vi "Polling.vi"(8 "error in (no error)":errorcluster, 11 "Node Ptr":T1 format="%.0x") -> (0 "error out":errorcluster)   [LabVIEW 2019, in "Diagnostics Addon System Explorer.lvlib"]
uses:
  Diagnostics Addon System Explorer.lvlib
  <vilib>/NI VeriStand/Custom Device API/Custom Device Item Ref.ctl
  Types/FG.Action.ctl
  Addon Shared/SubVIs/Constants.vi
  <vilib>/NI VeriStand/Custom Device API/Custom Device API.lvlib
panel:
  in  "SHDocVw.IWebBrowser":refnum<k7>(container)
  in  "Collection":i32(listbox) caption="Items"
  in  "Description":string
  out "Name":string
  in  "Header":cluster{"Section Name":string}={"Section Name"="Custom Device Item Settings"}
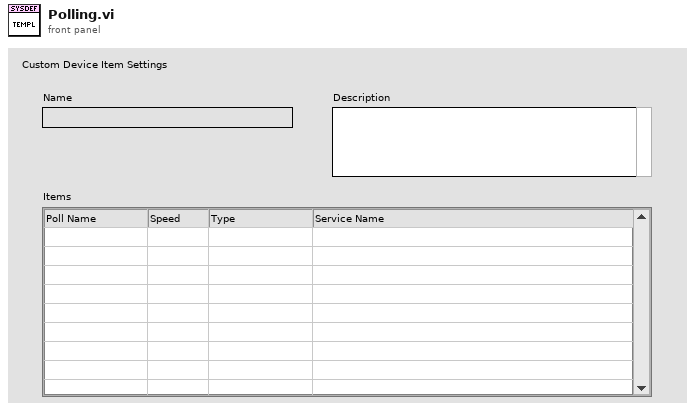
[diagram p1: front panel]
types:
  T1 = typedef "Custom Device API.lvlib/Custom Device Item Ref.ctl" = u64
  T2 = typedef "Diagnostics Addon System Explorer.lvlib/FG.Action.ctl" = enum16{"Get", "Set"}
  T3 = typedef "Custom Device API.lvlib/Custom Device Item Info.ctl" = cluster{"Name":string, "Is Channel":bool, "GUID":string, "Is Waveform":bool}
  T4 = typedef "Diagnostics Addon System Explorer.lvlib/Poll.Settings.ctl" = cluster{"Input Channels":T5[], "Speed":T6}
  T5 = typedef "Diagnostics Addon System Explorer.lvlib/Poll.LinkedNode.ctl" = cluster{"Node ID":u64}
  T6 = typedef "Diagnostics Addon Shared.lvlib/DPID.Rate.ctl" = enum16{"Slow", "Medium", "Fast"}
  T7 = typedef "Custom Device API.lvlib/Custom Device Commands.ctl" = enum16{"Default", "Item renamed", "Shutdown", "Dynamic button pressed"}
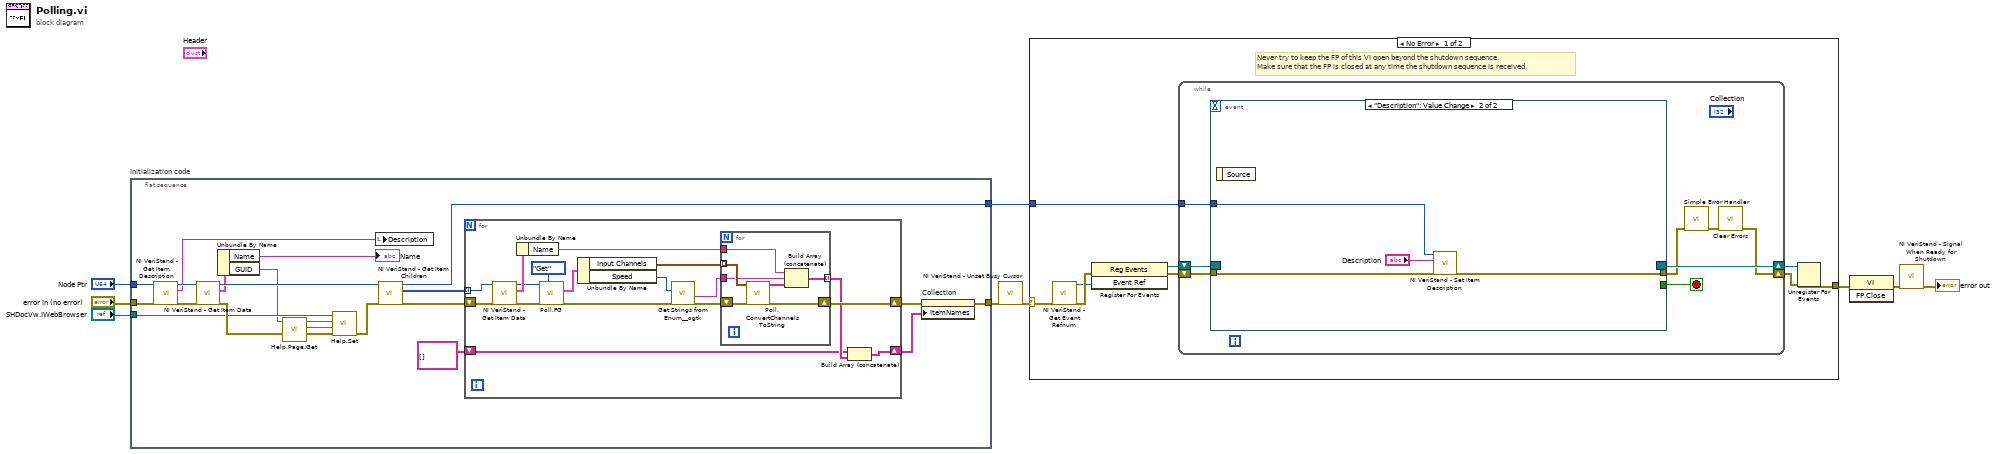
[diagram p0: block diagram]
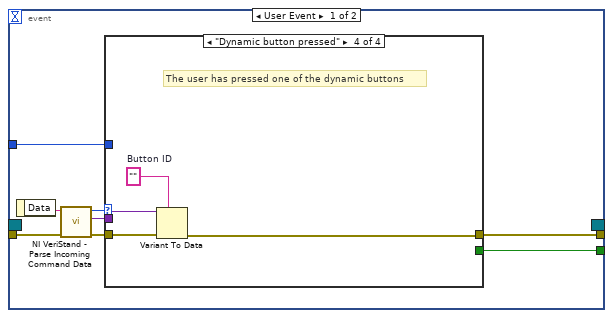
[diagram p2: hidden frame]
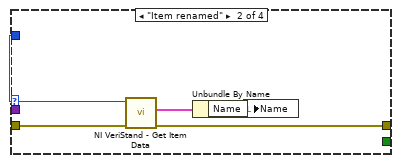
[diagram p4: hidden frame]
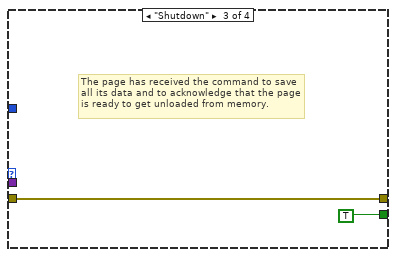
[diagram p5: hidden frame]
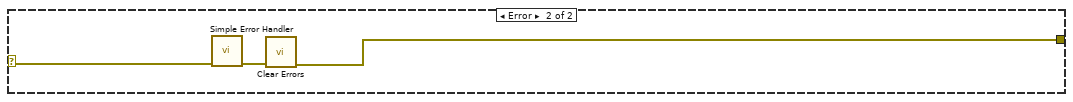
[diagram p6: hidden frame]
diagram:
  n1 = flat-sequence "Initialization code" {
    tunnel: "error in (no error)" -> [w15]
    tunnel: [w20] -> w6
    tunnel: [w22] -> w3
    tunnel: "Node Ptr" -> [w25]
    tunnel: "SHDocVw.IWebBrowser" -> [w16]
    frame #0 {
      n2 = call <vilib>:"NI VeriStand - Get Item Description.vi"("error in (no error)"=w15, "Item Ref in"=w25) -> ("error out"=w27:errorcluster, "Description"=w28:string, "Item Ref out"=w29:T1)  [unwired: 7 out]
      n3 = call <vilib>:"NI VeriStand - Get Item Data.vi"("error in (no error)"=w27, "Item Ref in"=w29) -> ("error out"=w18:errorcluster, "Item Info"=w26:T3, "Item Ref out"=w30:T1)  [unwired: 7 out]
      n4 = Unbundle By Name(w26) -> ("Name"=→"Name":string, "GUID"=w12:string)
      n5 = call "Help.Page.Get.vi"("GUID"=w12) -> ("HTML File"=w11:string, "Main CHM File"=w10:string)  [unwired: 9 in]
      n6 = call "Help.Set.vi"("error in (no error)"=w18, "HTML File"=w11, "Main CHM File"=w10, "SHDocVw.IWebBrowser2"=w16) -> ("error out"=w17:errorcluster)  [unwired: 7 in]
      n7 = local write "Description"(w28) -> ()
      n8 = call <vilib>:"NI VeriStand - Get Item Children.vi"("error in (no error)"=w17, "Item Ref in"=w30) -> ("error out"=w24:errorcluster, "Child Refs"=w23:T1[], "Item Ref out"=w22:T1)  [unwired: 6 in, 1 out]
      n9 = for {
        shift-right: [w40] -> w21
        shift-left: w24 -> [w46]
        tunnel: w23 -> [w45] mode=indexing
        shift-right: [w37] -> w14
        shift-left: string[][] [] -> [w36]
        n10 = call <vilib>:"NI VeriStand - Get Item Data.vi"("error in (no error)"=w46, "Item Ref in"=w45) -> ("error out"=w42:errorcluster, "Item Info"=w47:T3, "Item Ref out"=w41:T1)  [unwired: 7 out]
        n11 = Unbundle By Name(w47) -> ("Name"=w39:string)
        n12 = call "Poll.FG.vi"("Action"=FG.Action."Get", "error in"=w42, "Parent Ref"=w41) -> ("error out"=w35:errorcluster, "Selected Channels out"=w43:T4)  [unwired: 6 in, 1 out]
        n13 = Unbundle By Name(w43) -> ("Input Channels"=w31:T5[], "Speed"=w33:T6)
        n14 = call <userlib>:"Get Strings from Enum__ogtk.vi"("error in (no error)"=w35, "Enum"=w33) -> ("error out"=w34:errorcluster, "String Value"=w32:string)  [unwired: 6 in, 2 out]
        n15 = for {
          shift-right: [w52] -> w40
          shift-left: w34 -> [w54]
          tunnel: w31 -> [w53] mode=indexing
          tunnel: [w49] -> w38 mode=indexing
          tunnel: w39 -> [w51]
          tunnel: w32 -> [w48]
          n16 = call "Poll.ConvertChannelsToString.vi"("error in (no error)"=w54, "MonitoredChannelSettings"=w53) -> ("error out"=w52:errorcluster, "Array"=w50:string[])  [unwired: 8 in]
          n17 = Build Array (concatenate)(w51, w48, w50) -> (w49:string[])
        }
        n18 = Build Array (concatenate)(w36, w38) -> (w37:string[][])
      }
      n19 = property on="Collection" class="MCListbox (strict)"(error in=w21, "ItemNames"=w14) -> (error out=w20:errorcluster)  [unwired: 1 in, 1 out]
    }
  }
  n20 = call <vilib>:"NI VeriStand - Unset Busy Cursor.vi"("error in (no error)"=w6) -> ("error out"=w5:errorcluster)  [unwired: 10 out]
  n21 = case shown="No Error" w5 {
    selector: w5 -> [w55 w98]
    tunnel: [w60 w96] -> w9
    tunnel: w3 -> [w56 _]
    frame No Error {
      # "Never try to keep the FP of this VI open beyond the shutdown sequence.\nMake sure that the FP is closed at any time the shutdown sequence is received."
      n22 = call <vilib>:"NI VeriStand - Get Event Refnum.vi"("error in (no error)"=w55) -> ("error out"=w63:errorcluster, "Event Ref"=w59:refnum<user-event>)  [unwired: 9 out]
      n23 = register-events(error in=w63, w59) -> (reference out=w57:refnum<event-registration>, error out=w58:errorcluster)  [unwired: 1 in]
      n24 = while {
        tunnel: w56 -> [w67]
        shift-right: [w64] -> w61
        shift-left: w58 -> [w70]
        shift-right: [w71] -> w62
        shift-left: w57 -> [w69]
        stop <- w68 stop-if-true
        n25 = event shown="[1] \"Description\": Value Change" {
          selector: w69 -> [_ _]
          dyn-events: [_ _] -> w71
          timeout: _ -> [_ _]
          tunnel: w70 -> [w79 w94]
          tunnel: [w75 _] -> w68
          tunnel: [w74 w93] -> w66
          tunnel: w67 -> [w73 w95]
          event User Event {
            n26 = event-data() -> ("Data"=w78:string)  [unwired: 1 out]
            n27 = call <vilib>:"NI VeriStand - Parse Incoming Command Data.vi"("error in (no error)"=w79, "Incoming data"=w78) -> ("error out"=w77:errorcluster, "Outgoing data"=w72:variant, "Action"=w76:T7)  [unwired: 7 out]
            n28 = case shown="\"Dynamic button pressed\"" w76 {
              tunnel: w77 -> [w80 w85 w86 w91]
              tunnel: [_ _ TRUE _] -> w75
              tunnel: [w80 w82 w86 w88] -> w74
              tunnel: w73 -> [_ w84 _ _]
              tunnel: w72 -> [_ _ _ w90]
              frame "Default", Default {
              }
              frame "Item renamed" {
                n29 = call <vilib>:"NI VeriStand - Get Item Data.vi"("error in (no error)"=w85, "Item Ref in"=w84) -> ("error out"=w82:errorcluster, "Item Info"=w83:T3)  [unwired: 8 out]
                n30 = Unbundle By Name(w83) -> ("Name"=w81:string)
                n31 = local write "Name"(w81) -> ()
              }
              frame "Shutdown" {
                # "The page has received the command to save all its data and to acknowledge that the page is ready to get unloaded from memory."
              }
              frame "Dynamic button pressed" {
                w89 = ""  # Button ID
                # "The user has pressed one of the dynamic buttons"
                n32 = Variant To Data(error in=w91, type=w89, Variant=w90) -> (error out=w88:errorcluster)  [unwired: 1 out]
              }
            }
          }
          event "Description": Value Change {
            n33 = event-data() -> ()  [unwired: 2 out]
            n34 = call <vilib>:"NI VeriStand - Set Item Description.vi"("error in (no error)"=w94, "Description"="Description", "Item Ref in"=w95) -> ("error out"=w93:errorcluster)  [unwired: 8 out]
          }
        }
        n35 = call <vilib>:"Simple Error Handler.vi"("error in (no error)"=w66) -> ("error out"=w65:errorcluster)  [unwired: 1 in, 7 out]
        n36 = call <vilib>:"Clear Errors.vi"("error in (no error)"=w65) -> ("error out"=w64:errorcluster)  [unwired: 1 in, 5 out]
      }
      n37 = Unregister For Events(event registration refnum=w62, error in=w61) -> (error out=w60:errorcluster)
    }
    frame Error {
      n38 = call <vilib>:"Simple Error Handler.vi"("error in (no error)"=w98) -> ("error out"=w97:errorcluster)  [unwired: 1 in, 7 out]
      n39 = call <vilib>:"Clear Errors.vi"("error in (no error)"=w97) -> ("error out"=w96:errorcluster)  [unwired: 1 in, 5 out]
    }
  }
  n40 = invoke class="VI" method="FP.Close"(error in=w9) -> (error out=w8:errorcluster)  [unwired: 2 in, 2 out]
  n41 = call <vilib>:"NI VeriStand - Signal When Ready for Shutdown.vi"("error in (no error)"=w8) -> ("error out"=→"error out":errorcluster)  [unwired: 10 out]
